vi "GetTagsStringsAndValues.vi"() -> (3 "Strings And Values []":T1)   [LabVIEW 2019]
uses:
  <userlib>/TaikoLaser/PDLM_Tag.ctl
  <vilib>/Utility/miscctls.llb/LVStringsAndValuesArrayTypeDef_U32.ctl
panel:
  in  "Tag":T2 format="%x" items=["NONE"=0, "Locked"=16, "SoftLock"=17, "KeyLock"=18, "Class_IV_Lock"=20, "Interlock"=24, "LaserMode"=32, "LDH_PulsePowerTable"=33, "TriggerMode"=48, "TriggerLevelRaw"=64, "TriggerLevelRawLoLimit"=65, "TriggerLevelRawHiLimit"=66, "TriggerLevel"=72, "TriggerLevelLoLimit"=73, "TriggerLevelHiLimit"=74, "FastGate"=80, "FastGateImp"=96, "SlowGate"=112, "TargetTempRaw"=144, "TargetTempRawLoLimit"=145, "TargetTempRawHiLimit"=146, "CurrentTempRaw"=148, "CaseTempRaw"=149, "TargetTemp"=152, "TargetTempLoLimit"=153, "TargetTempHiLimit"=154, "CurrentTemp"=156, "CaseTemp"=157, "TempScale"=159, "Frequency"=168, "FrequencyLoLimit"=169, "FrequencyHiLimit"=170, "PulsePowerRaw"=176, "PulsePowerRawLoLimit"=177, "PulsePowerRawHiLimit"=178, "PulsePowerPermille"=180, "PulseShape"=181, "PulsePower"=184, "PulsePowerLoLimit"=185, "PulsePowerHiLimit"=186, "PulsePowerNanowatt"=188, "PulsePowerVoltage"=190, "PulseEnergy"=191, "CwPowerRaw"=192, "CwPowerRawLoLimit"=193, "CwPowerRawHiLimit"=194, "CwPowerPermille"=196, "CwPower"=200, "CwPowerLoLimit"=201, "CwPowerHiLimit"=202, "CwPowerMicroWatt"=204, "BurstLen"=208, "BurstPeriod"=224, "LDH_Fan"=240, "UI_Exclusive"=256]
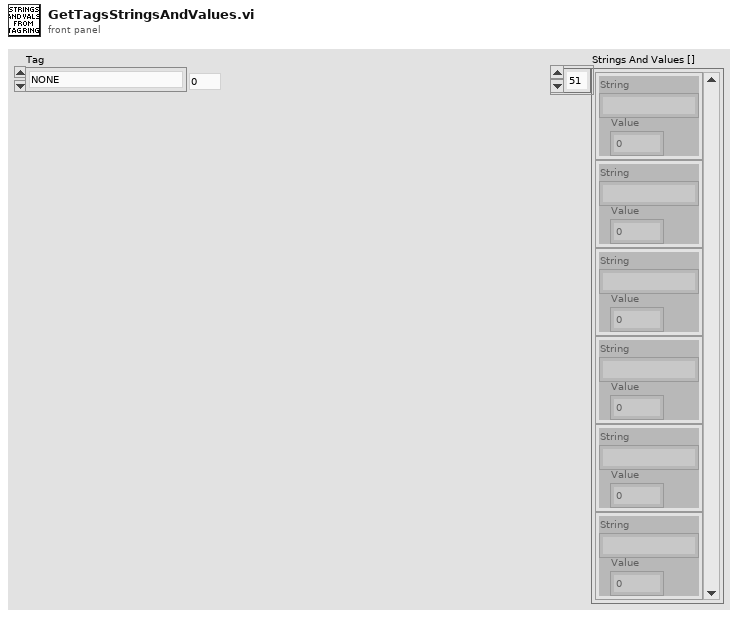
[diagram p1: front panel]
types:
  T1 = typedef "LVStringsAndValuesArrayTypeDef_U32.ctl" = cluster{"String":string, "Value":u32}[]
  T2 = typedef "PDLM_Tag.ctl" = u32
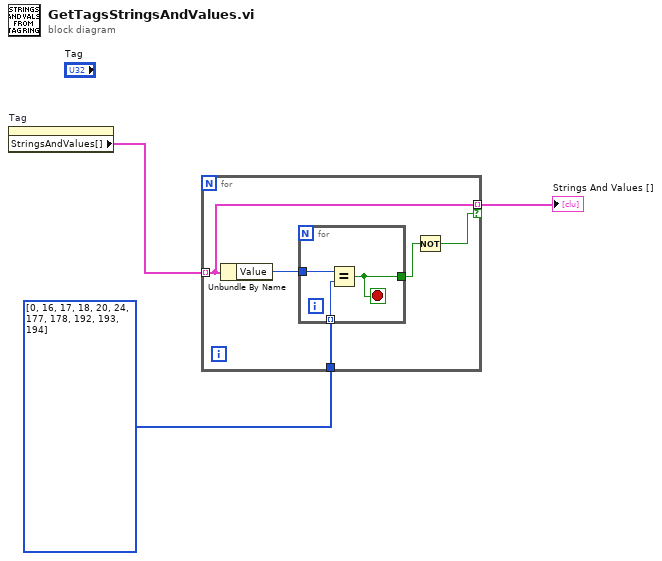
[diagram p0: block diagram]
diagram:
  n1 = property on="Tag" class="MDér (strict)"() -> ("StringsAndValues[]"=w3:T1)  [unwired: 2 in, 2 out]
  n2 = for {
    tunnel: w3 -> [w6] mode=indexing
    tunnel: u32[] [0, 16, 17, 18, 20, 24, 177, 178, 192, 193, 194] -> [w7]
    tunnel: [w6] -> w1 mode=indexing if=w4
    n3 = Unbundle By Name(w6) -> ("Value"=w8:u32)
    n4 = for {
      tunnel: w8 -> [w10]
      tunnel: w7 -> [w11] mode=indexing
      tunnel: [w9] -> w5
      stop <- w9 stop-if-true
      n5 = Equal?(x=w10, y=w11) -> (x = y?=w9:bool)
    }
    n6 = Not(x=w5) -> (.not. x?=w4:bool)
  }
  "Strings And Values []" <- w1
